vi "Pre Launch Init.vi"(11 "Nested in":refnum<class "Nested.lvclass">) -> (0 "error out":errorcluster, 3 "Nested out":refnum<class "Nested.lvclass">)   [LabVIEW 2020, in "Nested.lvlib" / "Nested.lvclass"]
doc: "(<B>Filename</B>: Actor Framework.lvlib:Actor.lvclass:Pre Launch Init.vi)\n\nDefines behavior that occurs after the Launch Nested Actor method is invoked but before the actor's Actor Core method begins running.\n\nBy default, this method does nothing. A descendant class may override it to define behavior."
uses:
  Nested.lvclass
  C:/Program Files/National Instruments/LabVIEW 2020/vi.lib/ActorFramework/Actor/Actor.lvclass
  Nested.lvclass/Nested.ctl
  <vilib>/ActorFramework/Actor/Actor.lvclass/Actor.ctl
  <vilib>/ActorFramework/Message Enqueuer/Message Enqueuer.lvclass/Message Enqueuer.ctl
  <vilib>/ActorFramework/Message Enqueuer/Init from Existing Queue.vi
  <vilib>/ActorFramework/Actor/Actor.lvclass
  <vilib>/ActorFramework/Message Enqueuer/Message Enqueuer.lvclass
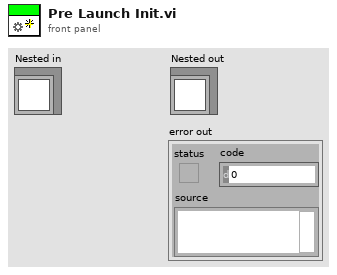
[diagram p1: front panel]
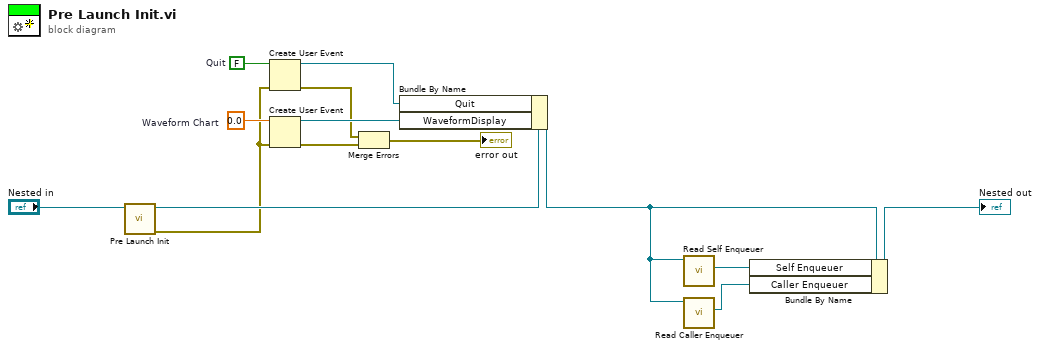
[diagram p0: block diagram]
diagram:
  w12 = FALSE  # Quit
  w11 = 0.0  # Waveform Chart
  n1 = call-parent "Pre Launch Init.vi"("Actor in"="Nested in") -> ("error out"=w8:errorcluster, "Actor out"=w14:refnum<class "Nested.lvclass">)  [unwired: 9 in]
  n2 = Create User Event(user event datatype=w12, error in=w8) -> (user event=w10:refnum<user-event>, error out=w7:errorcluster)
  n3 = Create User Event(user event datatype=w11, error in=w8) -> (user event=w9:refnum<user-event>, error out=w6:errorcluster)
  n4 = Merge Errors(w7, w6) -> (→"error out":errorcluster)
  n5 = Bundle By Name(cluster=w14, "Quit"=w10, "WaveformDisplay"=w9) -> (w4:refnum<class "Nested.lvclass">)
  n6 = call <vilib>:"Read Self Enqueuer.vi"("Actor"=w4) -> ("Self Enqueuer"=w2:refnum<class "Message Enqueuer.lvclass">)  [unwired: 10 in]
  n7 = call <vilib>:"Read Caller Enqueuer.vi"("Actor"=w4) -> ("Caller Enqueuer"=w1:refnum<class "Message Enqueuer.lvclass">)  [unwired: 10 in]
  n8 = Bundle By Name(cluster=w4, "Self Enqueuer"=w2, "Caller Enqueuer"=w1) -> (→"Nested out":refnum<class "Nested.lvclass">)
